vi "Get.vi"(11 "Timestamp in":refnum<class "Timestamp.lvclass">) -> (2 "Value":timestamp)   [LabVIEW 2020, in "Conditu2.lvlib" / "Columns.lvlib" / "Timestamp.lvclass"]
uses:
  Timestamp.lvclass
  Timestamp.lvclass/Timestamp.ctl
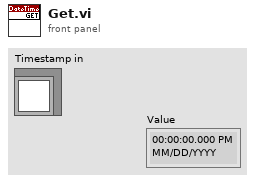
[diagram p1: front panel]
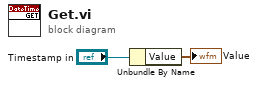
[diagram p0: block diagram]
diagram:
  n1 = Unbundle By Name("Timestamp in") -> ("Value"=→"Value":timestamp)
